vi "test_GPIB to RS-xxx ConvBox Initialize.vi"(8 "error in (no error)":errorcluster, 11 "TestCase in":refnum<class "Serial Protocols Tests.lvclass">) -> (0 "error out":errorcluster, 3 "TestCase out":refnum<class "Serial Protocols Tests.lvclass">)   [LabVIEW 2019, in "Serial Protocols Tests.lvclass"]
uses:
  Serial Protocols Tests.lvclass
  Listener/Listener.lvclass
  Listener/ListenerClassControls/Operation.ctl
  RS-xxx to GPIB ConvBox/RS-xxx to GPIB ConvBox.lvclass
  D:/GitRepository/niveristand-instrument-addon-classes/Source/Protocols/Protocol Parent/Protocol Parent.lvclass
  RS-xxx to GPIB ConvBox/RS-xxx to GPIB ConvBox.lvclass/RS-xxx to GPIB ConvBox.ctl
  RS-xxx to GPIB ConvBox/Data Access/Write IST bit sense.vi
  RS-xxx to GPIB ConvBox/Data Access/Write System controller.vi
  RS-xxx to GPIB ConvBox/Data Access/Write Assert Ren with IFC.vi
  RS-xxx to GPIB ConvBox/Data Access/Write ConvBox Address.vi
  RS-xxx to GPIB ConvBox/Data Access/Write Port.vi
  <vilib>/addons/_JKI Toolkits/VI Tester/TestCase.llb/TestCase.lvclass
  C:/Program Files (x86)/National Instruments/LabVIEW 2019/vi.lib/addons/_JKI Toolkits/VI Tester/TestCase.llb/TestCase.lvclass
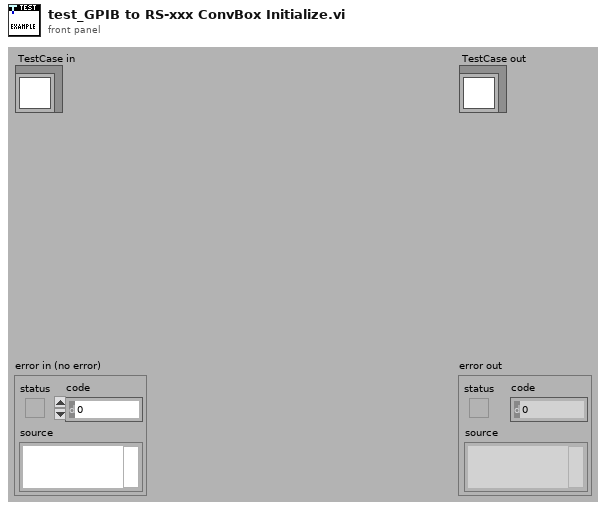
[diagram p1: front panel]
types:
  T1 = cluster{"IST Bit Sens":bool, "Assert Ren with IFC":bool, "system controller":bool}[]
  T2 = typedef "Listener.lvclass/Operation.ctl" = enum16{"Read", "Write"}
  T3 = typedef "Listener.lvclass/RS-xxx To GPIB ConvBox Data Structure.ctl" = cluster{"Protocol Port Ref":refnum<visa-resource-name>, "Listener Port Ref":refnum<visa-resource-name>, "Data":string, "Command Messages Read":string[], "Address":string}
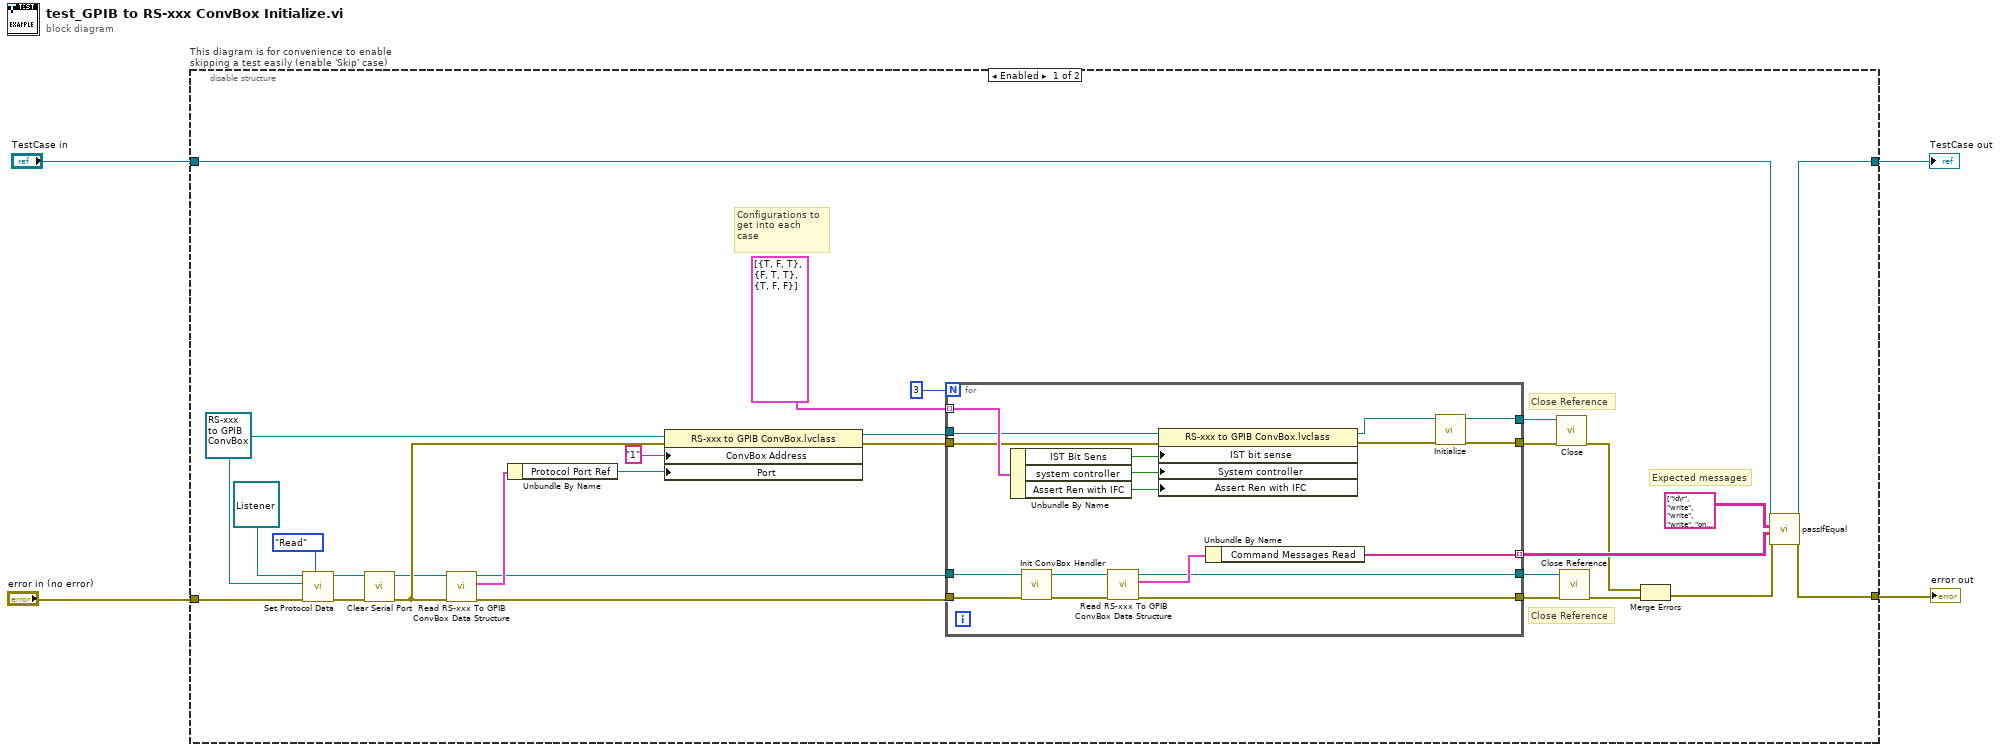
[diagram p0: block diagram]
diagram:
  n1 = disable-structure "This diagram is for convenience to enable skipping a test easily (enable 'Skip' case)" shown="Enabled" {
    disable-tunnel: "TestCase in" -> [w33 w55]
    disable-tunnel: [w11 w53] -> w1
    disable-tunnel: [w12 w54] -> w3
    disable-tunnel: "error in (no error)" -> [w30 w52]
    frame Enabled {
      w27 = refnum<class "RS-xxx to GPIB ConvBox.lvclass"> refnum ("Protocols.lvlib:RS-xxx to GPIB ConvBox.lvclass")
      # "Close Reference"
      # "Close Reference"
      # "Configurations to\nget into each \ncase"
      # "Expected messages"
      n2 = call "Set Protocol Data.vi"("Operation"=Operation."Read", "error in (no error)"=w30, "Protocols.lvlib:Protocol Parent.lvclass"=w27, "Listener In.lvclass"=refnum<class "Listener.lvclass"> refnum ("Listener.lvclass")) -> ("error out"=w26:errorcluster, "Listener Out.lvclass"=w25:refnum<class "Listener.lvclass">)  [unwired: 6 in]
      n3 = call "Clear Serial Port.vi"("error in (no error)"=w26, "Listener In.lvclass"=w25) -> ("error out"=w22:errorcluster, "Listener out"=w21:refnum<class "Listener.lvclass">)  [unwired: 8 in]
      n4 = call-dynamic "Read RS-xxx To GPIB ConvBox Data Structure.vi"("error in (no error)"=w22, "Listener in"=w21) -> ("error out"=w17:errorcluster, "RS-xxx To GPIB ConvBox Data Structure"=w24:T3, "Listener out"=w16:refnum<class "Listener.lvclass">)  [unwired: 7 in]
      n5 = Unbundle By Name(w24) -> ("Protocol Port Ref"=w23:refnum<visa-resource-name>)
      n6 = property class="RS-xxx to GPIB ConvBox.lvclass"(reference=w27, error in=w22, "ConvBox Address"="1", "Port"=w23) -> (reference out=w19:refnum<class "RS-xxx to GPIB ConvBox.lvclass">, error out=w18:errorcluster)
      n7 = for {
        N: 3 -> [_]
        tunnel: [w49] -> w5
        tunnel: [w45] -> w13 mode=indexing
        tunnel: T1 [{"IST Bit Sens"=TRUE, "Assert Ren with IFC"=FALSE, "system controller"=TRUE}, {"IST Bit Sens"=FALSE, "Assert Ren with IFC"=TRUE, "system controller"=TRUE}, {"IST Bit Sens"=TRUE, "Assert Ren with IFC"=FALSE, "system controller"=FALSE}] -> [w42] mode=indexing
        tunnel: w19 -> [w37]
        tunnel: w16 -> [w34]
        tunnel: [w44] -> w9
        tunnel: w17 -> [w35]
        tunnel: [w43] -> w10
        tunnel: w18 -> [w36]
        tunnel: [w38] -> w7
        n8 = Unbundle By Name(w42) -> ("IST Bit Sens"=w41:bool, "system controller"=w40:bool, "Assert Ren with IFC"=w39:bool)
        n9 = call "Init ConvBox Handler.vi"("error in (no error)"=w35, "Listener in"=w34) -> ("error out"=w47:errorcluster, "Listener out"=w48:refnum<class "Listener.lvclass">)  [unwired: 8 in]
        n10 = call-dynamic "Read RS-xxx To GPIB ConvBox Data Structure.vi"("error in (no error)"=w47, "Listener in"=w48) -> ("error out"=w43:errorcluster, "RS-xxx To GPIB ConvBox Data Structure"=w46:T3, "Listener out"=w44:refnum<class "Listener.lvclass">)  [unwired: 7 in]
        n11 = property class="RS-xxx to GPIB ConvBox.lvclass"(reference=w37, error in=w36, "IST bit sense"=w41, "System controller"=w40, "Assert Ren with IFC"=w39) -> (reference out=w50:refnum<class "RS-xxx to GPIB ConvBox.lvclass">, error out=w51:errorcluster)
        n12 = Unbundle By Name(w46) -> ("Command Messages Read"=w45:string[])
        n13 = call-dynamic "Initialize.vi"("error in (no error)"=w51, "RS232 to GPIB ConvBox in"=w50) -> ("error out"=w38:errorcluster, "RS232 to GPIB ConvBox out"=w49:refnum<class "RS-xxx to GPIB ConvBox.lvclass">)  [unwired: 8 in]
      }
      n14 = call-dynamic "Close.vi"("error in (no error)"=w7, "RS232 to GPIB ConvBox in"=w5) -> ("error out"=w6:errorcluster)  [unwired: 8 in, 1 out]
      n15 = call "Close Reference.vi"("error in (no error)"=w10, "Listener In.lvclass"=w9) -> ("error out"=w8:errorcluster)  [unwired: 9 in]
      n16 = Merge Errors(w6, w8) -> (w29:errorcluster)
      n17 = call-dynamic "passIfEqual.vi"("error in (no error)"=w29, "y"=w13, "x"=string[][] [["id\r", "write", "write", "write", "onl 1\r", "caddr 1\r", "sic\r", "eos D\r", "eot 1\r", "rsc 1\r", "sre 0\r", "ist 1\r", "tmo 1,1\r"], ["id\r", "write", "write", "write", "onl 1\r", "caddr 1\r", "rsc 1\r", "sre 1\r", "tmo 1,1\r", "", "", "", ""], ["id\r", "write", "write", "write", "onl 1\r", "caddr 1\r", "rsc 0\r", "ist 1\r", "tmo 1,1\r", "", "", "", ""]] ("Command Messages Read"), "TestCase in"=w33) -> ("error out"=w12:errorcluster, "TestCase out"=w11:refnum<class "Serial Protocols Tests.lvclass">)  [unwired: 6 in]
    }
    frame Disabled {
      # "skip test result while test is under development"
      n18 = call <vilib>:"skip.vi"("error in (no error)"=w52, "TestCase in"=w55) -> ("error out"=w54:errorcluster, "TestCase out"=w53:refnum<class "Serial Protocols Tests.lvclass">)  [unwired: 8 in]
    }
  }
  "error out" <- w3
  "TestCase out" <- w1
